vi "Pre Launch Init.vi"(11 "NI_DAQmx(AI) in":refnum<class "NI_DAQmx(AI).lvclass">) -> (0 "error out":errorcluster, 3 "NI_DAQmx(AI) out":refnum<class "NI_DAQmx(AI).lvclass">)   [LabVIEW 2025, in "NI_DAQmx(AI).lvclass"]
doc: "<p>(<strong>Filename</strong>: <span class=\"dnl\">Actor Framework.lvlib:Actor.lvclass:Pre Launch Init.vi</span>)</p>\n<p>Defines behavior that occurs after the <a href=\"nihelplauncher://docs/csh?context=lvcore_lvcomm_af_launch_nested_actor\">Launch Nested Actor</a> method is invoked but before the actor's Actor Core method begins running.</p>\n<p>By default, this method does nothing. A descendant class may override it to define behavior.</p>"
uses:
  NI_DAQmx(AI).lvclass
  NI_DAQmx(AI).lvclass/NI_DAQmx(AI).ctl
  Write task.vi
  <vilib>/DAQmx/create/channels.llb/DAQmx Create Channel (AI-Voltage-Basic).vi
  <vilib>/DAQmx/configure/timing.llb/DAQmx Timing (Sample Clock).vi
  DAQ_Abstr/Task_Type/AI_Task/AI_Task/AI_Task.lvclass
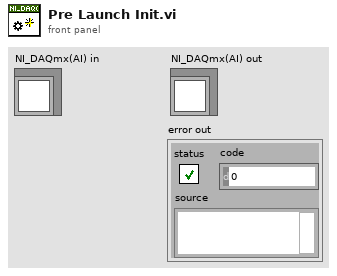
[diagram p1: front panel]
types:
  T1 = typedef "DAQ_Module.lvlib/DAQ_Module.lvclass/DAQ_Task_Config.ctl" = cluster{"TaskType":T2, "PhysicalChannels":string, "SampleRateConfiguration":cluster{"SampleRate":dbl, "SamplesPerChannel":u32, "SamplesPerRead":i32, "SampleMode":i32, "Clock Source":string}, "ChannelConfig":string}
  T2 = typedef "DAQ_Module.lvlib/DAQ_Module.lvclass/DAQ_Task_Type.ctl" = enum16{"AI", "Linear", "Angular", "AO"}
  T3 = typedef "DAQ_Module.lvlib/DAQ_Module.lvclass/DAQ_AI_Task_Config.ctl" = cluster{"MaxValue":dbl, "MinValue":dbl, "InputTerminalConfiguration":i32}
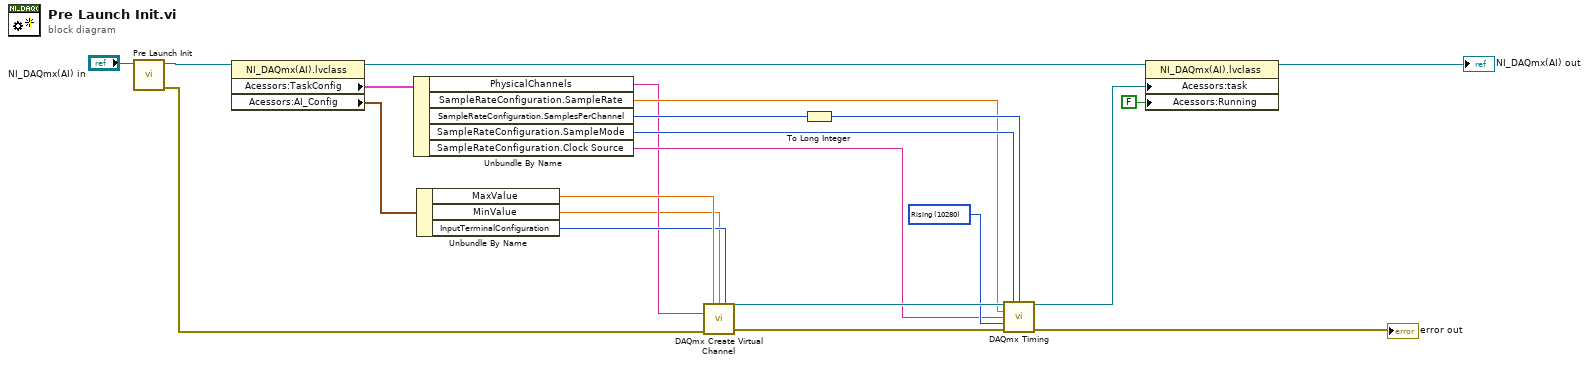
[diagram p0: block diagram]
diagram:
  w7 = 10280 items=["Rising"=10280, "Falling"=10171] ("active edge")
  n1 = call-parent "Pre Launch Init.vi"("Task_Abstr in"="NI_DAQmx(AI) in") -> ("error out"=w19:errorcluster, "Task_Abstr out"=w22:refnum<class "NI_DAQmx(AI).lvclass">)  [unwired: 9 in]
  n2 = property class="NI_DAQmx(AI).lvclass"(reference=w22) -> (reference out=w20:refnum<class "NI_DAQmx(AI).lvclass">, "Acessors:TaskConfig"=w14:T1, "Acessors:AI_Config"=w15:T3)  [unwired: 1 in, 1 out]
  n3 = Unbundle By Name(w14) -> ("PhysicalChannels"=w3:string, "SampleRateConfiguration.SampleRate"=w8:dbl, "SampleRateConfiguration.SamplesPerChannel"=w10:u32, "SampleRateConfiguration.SampleMode"=w11:i32, "SampleRateConfiguration.Clock Source"=w6:string)
  n4 = Unbundle By Name(w15) -> ("MaxValue"=w13:dbl, "MinValue"=w2:dbl, "InputTerminalConfiguration"=w12:i32)
  n5 = call-poly <vilib>:"DAQmx Create Virtual Channel.vi"("maximum value"=w13, "minimum value"=w2, "input terminal configuration"=w12, "physical channels"=w3, "error in"=w19) -> ("task out"=w16:refnum<k21>, "error out"=w18:errorcluster)  [unwired: 9 in]
  n6 = To Long Integer(number=w10) -> (32bit integer=w9:i32)
  n7 = call-poly <vilib>:"DAQmx Timing.vi"("task/channels in"=w16, "sample mode"=w11, "samples per channel"=w9, "rate"=w8, "source"=w6, "active edge"=w7, "error in"=w18) -> ("task out"=w4:refnum<k21>, "error out"=→"error out":errorcluster)  [unwired: 7 in]
  n8 = property class="NI_DAQmx(AI).lvclass"(reference=w20, "Acessors:task"=w4, "Acessors:Running"=FALSE ("Running")) -> (reference out=→"NI_DAQmx(AI) out":refnum<class "NI_DAQmx(AI).lvclass">)  [unwired: 1 in, 1 out]
